vi "Subvi DO.vi"(2 "DO channel":refnum<k21>="Connector1/DIO0", 8 "Ext trig enable":bool, 10 "Memory label":refnum<k21>="DO0 buffer") -> ()   [LabVIEW 2017]
uses:
  <vilib>/Platform/TimedLoop/XDataNode/timing_clust.ctl
  <vilib>/Platform/TimedLoop/XDataNode/nitl_modes.ctl
  <vilib>/Platform/TimedLoop/XDataNode/wakeup.ctl
  <vilib>/rvi/Emulation/niFpgaSctlEmulationGetInTimedLoop.vi
  <vilib>/rvi/Emulation/niFpgaEmulationReportErrorSimple.vi
  <vilib>/rvi/Emulation/niFpgaGetClockAttributes.vi
  <vilib>/rvi/Emulation/niFpgaCriticalErrorInLSC.vi
  Control/GV DO delay.vi
  Detector/GV line clock start.vi
  <vilib>/rvi/DataTransferAndStorage/Container/Common/niFpgaContainerExecOnDevCompGetState.vi
  <vilib>/rvi/Emulation/niFpgaEmulationIsFPGAContextNoSignature.vi
  <vilib>/rvi/DataTransferAndStorage/Container/Common/niFpgaContainerGetUniqueNameForEmu.vi
  <vilib>/rvi/Emulation/niFpgaProcessEmulError.vi
  <vilib>/rvi/errors/nirviReportUnexpectedCaseInternalError (U32).vi
  <vilib>/rvi/Memory/Memory_Emulation/niFpgaMemoryEmulationCacheClearOnFirstRun.vi
  <vilib>/rvi/Memory/Memory_Emulation/nirvimemoryEmulationManagerCache_MakeExclusive.vi
  <vilib>/rvi/Memory/Memory_Emulation/niFpgaMemoryEmulationValidateCache.vi
  <vilib>/rvi/Memory/Memory_Emulation/nirvimemoryEmulationManagerCache_InsertValue.vi
  <vilib>/Utility/error.llb/Clear Errors.vi
  <vilib>/rvi/Memory/Memory_Emulation/nirvimemoryEmulationManagerCache_ReleaseExclusive.vi
  <vilib>/rvi/Memory/Memory_Emulation/nirvimemoryEmulationManagerCache_GetValue.vi
  <vilib>/rvi/Memory/Memory_Emulation/nirvimemoryEmulationManagerCache_SetValue.vi
  <vilib>/rvi/Emulation/niFpgaSctlEmulationResourceMgr.vi
  <vilib>/rvi/eio/common/nirviEmuTemplateMethod_errors.vi
  <vilib>/Platform/TimedLoop/XDataNode/XDataNode.xnode
  <vilib>/rvi/DataTransferAndStorage/Container/XNode/niFpgaContainer.xnode
  <vilib>/rvi/Memory/Memory_Emulation/niFpgaMemoryEmulationRefIn.vi
  <vilib>/eio/EIONode/EIONode.xnode
  <vilib>/Platform/TimedLoop/XDataNode/XDNodeRunTimeDep.lvlib
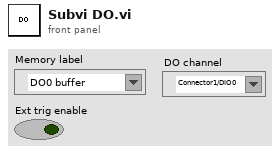
[diagram p1: front panel]
types:
  T1 = typedef "XDNodeRunTimeDep.lvlib/timing_clust.ctl" = cluster{"Expected End [f-1]":u64, "Actual End [f-1]":u64, "Finished Late? [f-1]":bool, "Expected End [i-1]":u64, "Actual End [i-1]":u64, "Finished Late? [i-1]":bool, "Expected Start [i]":u64, "Actual Start [i]":u64, "Expected Start [f]":u64, "Actual Start [f]":u64, "Source Name":string, "Structure Name":string, "Period":i64, "Deadline":i64, "Offset":i64, "Start":i64, "Priority":i32, "Timeout":i32, "Mode":T2, "Wakeup Reason":T3, "Error":errorcluster, "Source Type":string, "Secondary Source Type":string, "Global End Time":u64, "Global Start Time":u64, "Frame Duration":u64, "Iteration Duration":u64, "Assigned CPU":i32, "I/O Scan Engine Mode":u32}
  T2 = typedef "XDNodeRunTimeDep.lvlib/nitl_modes.ctl" = enum32{"No Change", "Process missed periods, maintain original phase", "Discard missed periods, maintain original phase", "Process missed periods, ignore original phase", "Discard missed periods, ignore original phase"}
  T3 = typedef "XDNodeRunTimeDep.lvlib/wakeup.ctl" = enum32{"Normal", "Aborted", "Asynchronous wakeup", "Timing source error", "Timed loop error", "Timeout"}
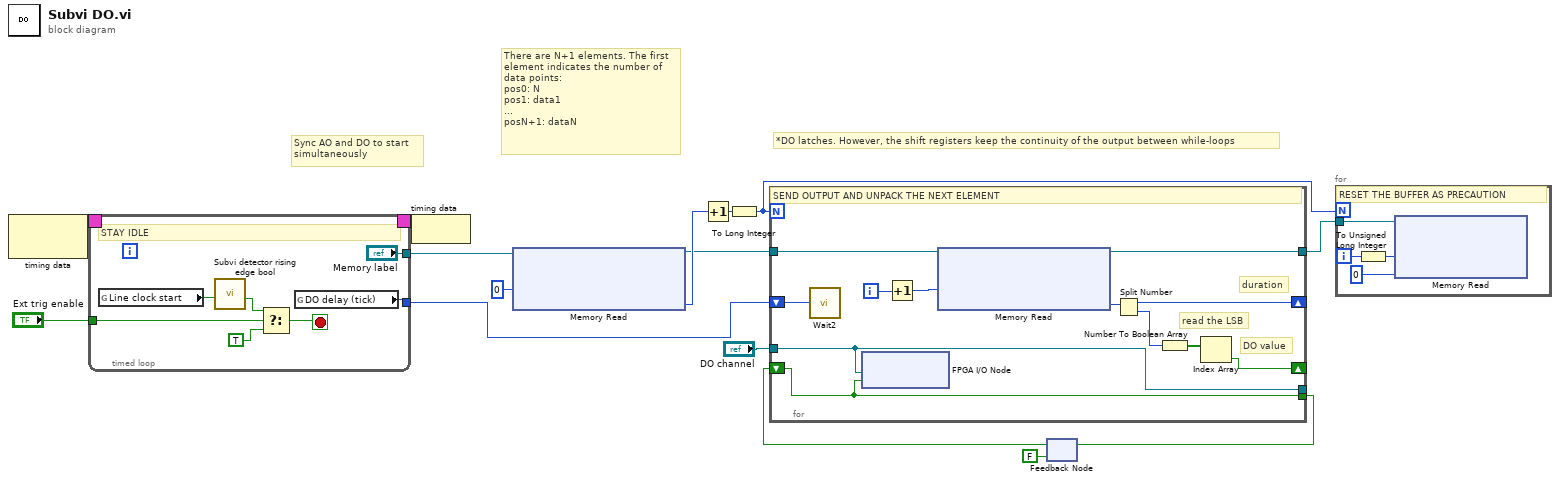
[diagram p0: block diagram]
diagram:
  # "There are N+1 elements. The first\nelement indicates the number of\ndata points:\npos0: N\npos1: data1\n...\nposN+1: dataN"
  # "*DO latches. However, the shift registers keep the continuity of the output between while-loops"
  # "Sync AO and DO to start\nsimultaneously"
  n1 = node-c288() -> (w5:T1)  [unwired: 1 in]
  n2 = timed-loop {
    tunnel: ["Memory label"] -> w3
    timing: w5 -> [_]
    timing-out: [_] -> w4
    tunnel: [w21] -> w2
    tunnel: "Ext trig enable" -> [w16]
    stop <- w19 stop-if-true
    # "STAY IDLE"
    n3 = global read "GV line clock start.vi" "Line clock start"() -> (w20:bool)
    n4 = call "Subvi detector rising edge bool.vi"("Input"=w20) -> ("Output"=w17:bool)  [unwired: 10 in]
    n5 = Select(t=w17, s=w16, f=TRUE) -> (s? t:f=w19:bool)
    n6 = global read "GV DO delay.vi" "DO delay (tick)"() -> (w21:u16)
  }
  n7 = node-c288(w4) -> ()
  n8 = xnode ("Memory Read")("Memory In"=w3, "Address"=u32 0) -> ("Memory Out"=w11:refnum<k21>, "Data"=w13:u32)
  n9 = Increment(x=w13) -> (x+1=w12:u32)
  n10 = To Long Integer(number=w12) -> (32bit integer=w10:i32)
  n11 = feedback #1(FALSE) -> (w8:bool)
  n12 = for {
    N: w10 -> [_]
    shift-right: [w31] -> _
    shift-left: w8 -> [w26]
    shift-right: [w33] -> _
    shift-left: w2 -> [w32]
    tunnel: [w30] -> w14
    tunnel: w11 -> [w29]
    tunnel: [w26] -> w6
    tunnel: "DO channel" -> [w25]
    tunnel: [w25] -> _
    i -> [w28]
    # "read the LSB"
    # "DO value"
    # "duration"
    # "SEND OUTPUT AND UNPACK THE NEXT ELEMENT"
    n13 = call "Wait2"("Count(Ticks)"=w32) -> ()  [unwired: 1 out]
    n14 = xnode "FPGA I/O Node"("I/O Item"=w26, "FPGA I/O In"=w25) -> ()  [unwired: 1 out]
    n15 = Increment(x=w28) -> (x+1=w27:i32)
    n16 = xnode ("Memory Read")("Address"=w27, "Memory In"=w29) -> ("Data"=w35:u32, "Memory Out"=w30:refnum<k21>)
    n17 = Split Number(x=w35) -> (hi(x)=w33:u16, lo(x)=w34:u16)
    n18 = Number To Boolean Array(number=w34) -> (Boolean array=w36:bool[])
    n19 = Index Array(array=w36) -> (element=w31:bool)  [unwired: 1 in]
  }
  n20 = feedback-in #1(w6) -> ()
  n21 = for {
    N: w10 -> [_]
    tunnel: w14 -> [w40]
    i -> [w39]
    # "RESET THE BUFFER AS PRECAUTION"
    n22 = To Unsigned Long Integer(number=w39) -> (unsigned 32bit integer=w37:u32)
    n23 = xnode ("Memory Read")("Address"=w37, "Data"=u32 0, "Memory In"=w40) -> ()  [unwired: 1 out]
  }
